vi "read_data2.vi"(8 "error in (no error)":errorcluster, 11 "GenericDAQ in":refnum<class "GenericDAQ.lvclass">) -> (0 "error out":errorcluster, 3 "GenericDAQ out":refnum<class "GenericDAQ.lvclass">)   [LabVIEW 2010, in "GenericDAQ.lvclass"]
uses:
  GenericDAQ.lvclass
  GenericDAQ.lvclass/GenericDAQ.ctl
  common/classes/GenericComponent/GenericComponent/class_data.vi
  common/classes/ErrorController/ErrorController/class_data.vi
  common/classes/GenericComponent/GenericComponent/GenericComponent.lvclass
  common/classes/ErrorController/ErrorController/ErrorController.lvclass
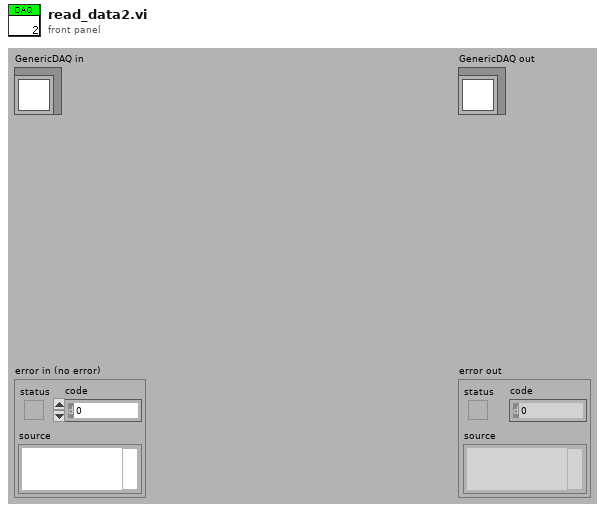
[diagram p1: front panel]
types:
  T1 = typedef "pixel_raw_data_array.ctl" = dbl[][]
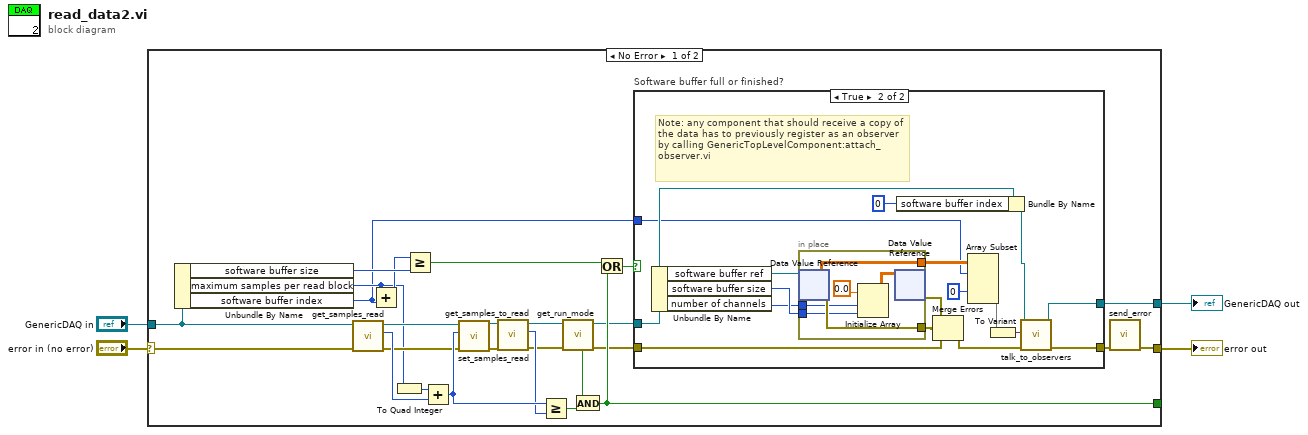
[diagram p0: block diagram]
diagram:
  n1 = case shown="No Error" "error in (no error)" {
    selector: "error in (no error)" -> [w30 w57]
    tunnel: [w11 w57] -> w2
    tunnel: [w22 w56] -> w1
    tunnel: "GenericDAQ in" -> [w13 w56]
    tunnel: [w20 _] -> _
    frame No Error {
      n2 = Unbundle By Name(w13) -> ("software buffer size"=w21:i32, "maximum samples per read block"=w6:i32, "software buffer index"=w5:i32)
      n3 = call-dynamic "get_samples_read.vi"("error in (no error)"=w30, "GenericDAQ.lvclass in"=w13) -> ("error out"=w9:errorcluster, "samples read"=w25:i64, "GenericDAQ.lvclass out"=w8:refnum<class "GenericDAQ.lvclass">)  [unwired: 7 out]
      n4 = Add(x=w6, y=w5) -> (x+y=w7:i32)
      n5 = To Quad Integer(1:w6) -> (0:w26:i64)
      n6 = Greater Or Equal?(x=w7, y=w21) -> (x >= y?=w19:bool)
      n7 = Add(x=w26, y=w25) -> (x+y=w27:i64)
      n8 = call-dynamic "set_samples_read.vi"("error in (no error)"=w9, "samples read"=w27, "GenericDAQ.lvclass in"=w8) -> ("error out"=w29:errorcluster, "GenericDAQ.lvclass out"=w28:refnum<class "GenericDAQ.lvclass">)  [unwired: 7 out]
      n9 = call-dynamic "get_samples_to_read.vi"("error in (no error)"=w29, "GenericDAQ.lvclass in"=w28) -> ("error out"=w17:errorcluster, "samples to read"=w24:i64, "GenericDAQ.lvclass out"=w15:refnum<class "GenericDAQ.lvclass">)  [unwired: 7 out]
      n10 = Greater Or Equal?(x=w27, y=w24) -> (x >= y?=w23:bool)
      n11 = call "get_run_mode.vi"("error in (no error)"=w17, "GenericPlugin in"=w15) -> ("error out"=w16:errorcluster, "GenericPlugin out"=w12:refnum<class "GenericDAQ.lvclass">, "is NOT free run?"=w14:bool)  [unwired: 5 in, 2 out]
      n12 = And(x=w14, y=w23) -> (x .and. y?=w20:bool)
      n13 = Or(x=w19, y=w20) -> (x .or. y?=w18:bool)
      n14 = case "Software buffer full or finished?" shown="True" w18 {
        tunnel: w16 -> [w32 w41]
        tunnel: [w32 w44] -> w10
        tunnel: [w31 w40] -> w22
        tunnel: w12 -> [w31 w39]
        tunnel: w5 -> [_ w34]
        frame False {
        }
        frame True {
          # "Note: any component that should receive a copy of the data has to previously register as an observer by calling GenericTopLevelComponent:attach_observer.vi"
          n15 = Unbundle By Name(w39) -> ("software buffer ref"=w48:refnum<data-value>, "software buffer size"=w43:i32, "number of channels"=w42:i32)
          n16 = in-place {
            in-place-border: [w55] -> w46
            in-place-border: [w54] -> w36
            in-place-border: w43 -> [w52]
            in-place-border: w42 -> [w51]
            n17 = in-place-dvr #1(w48) -> (w54:T1, w55:errorcluster)
            n18 = Initialize Array(0.0, w51, w52) -> (w50:dbl[][])
            n19 = in-place-dvr #1(w50) -> (w47:errorcluster)  [unwired: 1 out]
          }
          n20 = Bundle By Name(cluster=w39, "software buffer index"=0) -> (w38:refnum<class "GenericDAQ.lvclass">)
          n21 = Merge Errors(w47, w46, w41) -> (w45:errorcluster)
          n22 = Array Subset(array=w36, index (col)=0 ("index"), length (col)=w34) -> (w33:T1)  [unwired: 2 in]
          n23 = To Variant(anything=w33) -> (Variant=w49:variant)
          n24 = call-dynamic "talk_to_observers.vi"("error in (no error)"=w45, "data"=w49, "GenericToplevelComponent in"=w38) -> ("error out"=w44:errorcluster, "GenericToplevelComponent out"=w40:refnum<class "GenericDAQ.lvclass">)  [unwired: 7 in]
        }
      }
      n25 = call "send_error.vi"("error in (no error)"=w10) -> ("error out"=w11:errorcluster)  [unwired: 10 in]
    }
    frame Error {
    }
  }
  "error out" <- w2
  "GenericDAQ out" <- w1
